vi "Keep  Distance(SubVI).vi"(8 "Linear Gain":dbl=1.0, 9 "DC estimate (V)":dbl, 10 "AC estimate (Vrms)":dbl, 11 "desire(cm)":dbl) -> (1 "Linear_Array":dbl[](array[numeric]), 3 "goat":bool)   [LabVIEW 2019]
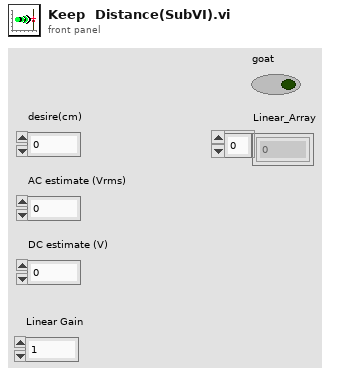
[diagram p1: front panel]
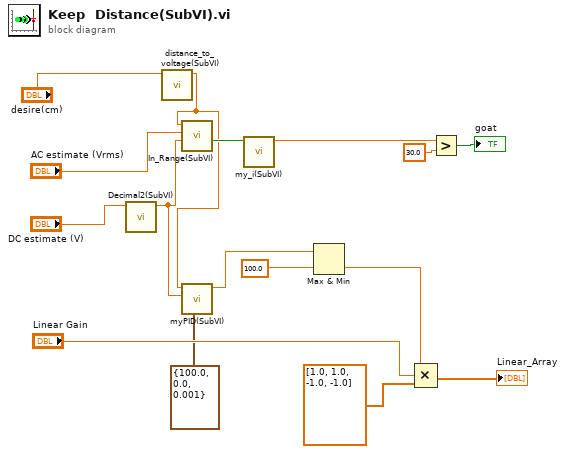
[diagram p0: block diagram]
diagram:
  n1 = call "Decimal2(SubVI).vi"("DC estimate (V)"="DC estimate (V)") -> ("Numeric"=w13:dbl)  [unwired: 10 in]
  n2 = call "distance_to_voltage(SubVI).vi"("distance(cm)"="desire(cm)") -> ("Voltage(V)"=w1:dbl)  [unwired: 10 in]
  n3 = call "In_Range(SubVI).vi"("Proccess Variable"=w13, "AC estimate (Vrms)"="AC estimate (Vrms)", "Setpoint"=w1) -> ("In Range?"=w7:bool)  [unwired: 7 in, 1 out]
  n4 = call "myPID(SubVI).vi"("Cluster"=cluster{"Kp":dbl, "Ki":dbl, "Kd":dbl} {"Kp"=100.0, "Ki"=0.0, "Kd"=0.001} ("parameter"), "Proccess Variable"=w13, "Setpoint"=w1) -> ("Speed(+-100%)"=w10:dbl)  [unwired: 8 in]
  n5 = call "my_i(SubVI).vi"("start"=w7) -> ("my_i"=w2:dbl)  [unwired: 9 in, 1 out]
  n6 = Max & Min(x=w10, y=100.0) -> (min(x,y)=w14:dbl)  [unwired: 1 out]
  n7 = Compound Arithmetic op=MULTIPLY(w14, "Linear Gain", dbl[] [1.0, 1.0, -1.0, -1.0]) -> (→"Linear_Array":dbl[])
  n8 = Greater?(x=w2, y=30.0) -> (0:→"goat":bool)
